vi "Configure Bus.vi"(4 "Digital Channel List":bool[](array[boolean]), 5 "Enable Bus (T: Enable)":bool=TRUE, 6 "Slope (0: Rising)":i32(ring) items=["Rising", "Falling", "Either"], 7 "Bus (51: Bus 1)":i32(ring)=51 items=["Bus 1"=51, "Bus 2"=52, "Bus 3"=53, "Bus 4"=54], 8 "error in (no error)":errorcluster, 9 "Clock Source (19: None)":i32(ring)=19 items=["Channel 1"=1, "Channel 2"=2, "Channel 3"=3, "Channel 4"=4, "DIG 0"=20, "DIG 1"=21, "DIG 2"=22, "DIG 3"=23, "DIG 4"=24, "DIG 5"=25, "DIG 6"=26, "DIG 7"=27, "DIG 8"=28, "DIG 9"=29, "DIG 10"=30, "DIG 11"=31, "DIG 12"=32, "DIG 13"=33, "DIG 14"=34, "DIG 15"=35, "None"=19], 10 "Bus Type (4: XAUI)":i32(ring)=4 items=["Can", "Fibre Channel", "SATA", "SPI", "XAUI", "Flex Ray", "GEN8B10B", "Generic", "IIC", "Infinite Band", "Most", "PCI Express", "SAS", "Hot Link", "MIPI", "DVI", "USB2", "USB3", "UART", "PCI3", "MPHY", "LIN", "JTAG", "GEN8B10B ", "E10GBASEKR", "DDR", "RFFE", "SVID", "CSI3", "Dig Rf", "JESD204B", "LLI", "SSIC", "UFS", "UNI Pro"], 11 "VISA resource name":refnum<visa-resource-name>) -> (0 "error out":errorcluster, 3 "VISA resource name out":refnum<visa-resource-name>)   [LabVIEW 2020, in "Agilent 90000 Series.lvlib"]
doc: "Configures the BUS settings in serial data analysis."
uses:
  Agilent 90000 Series.lvlib
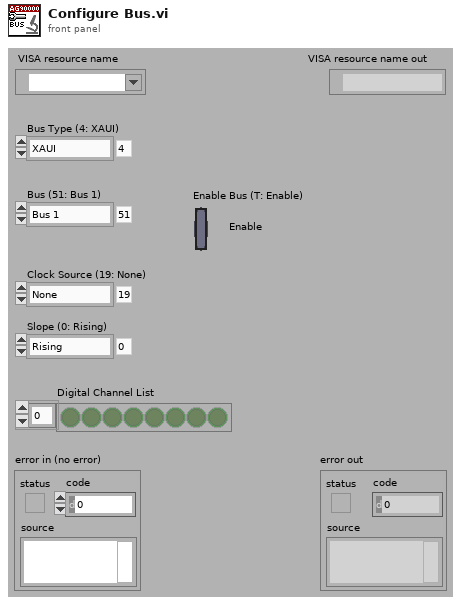
[diagram p1: front panel]
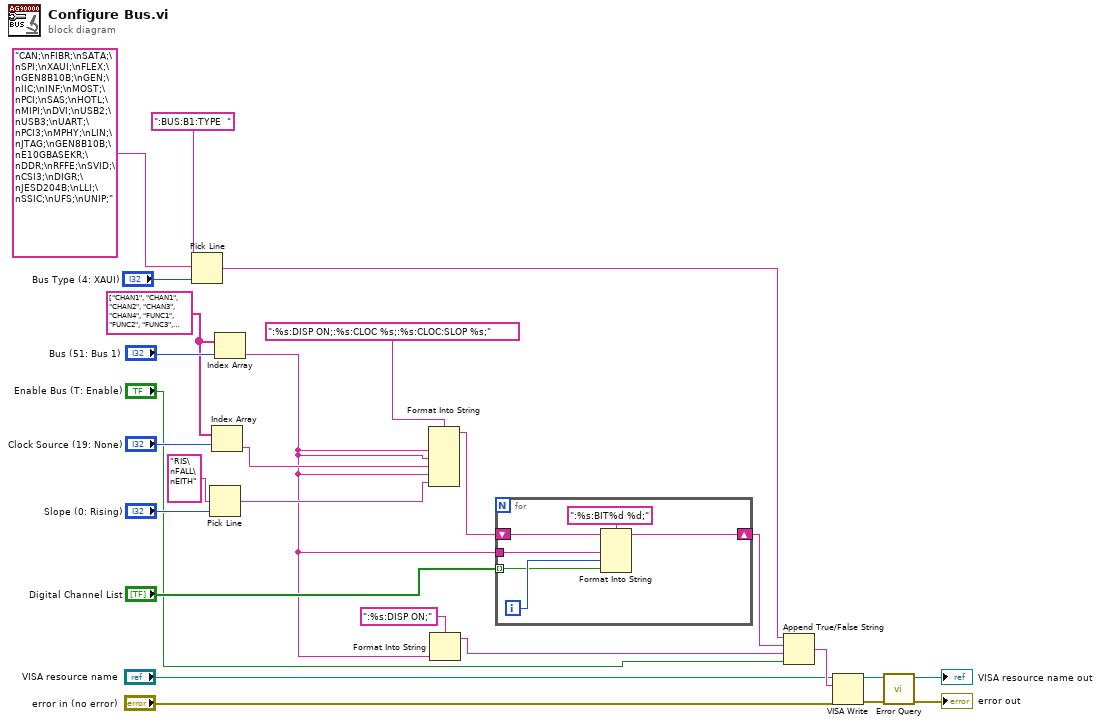
[diagram p0: block diagram]
diagram:
  w17 = string[] ["CHAN1", "CHAN1", "CHAN2", "CHAN3", "CHAN4", "FUNC1", "FUNC2", "FUNC3", "FUNC4", "WMEM1", "WMEM2", "WMEM3", "WMEM4", "AUX", "LINE", "CLOC", "MTR", "MSP", "EQU", "NONE", "DIG0", "DIG1", "DIG2", "DIG3", "DIG4", "DIG5", "DIG6", "DIG7", "DIG8", "DIG9", "DIG10", "DIG11", "DIG12", "DIG13", "DIG14", "DIG15", "", "", "", "", "", "POD1", "POD2", "", "", "", "", "", "", "", "", "BUS1", "BUS2", "BUS3", "BUS4"]
  n1 = Pick Line(string ("")=":BUS:B1:TYPE  ", multi-line string="CAN;\nFIBR;\nSATA;\nSPI;\nXAUI;\nFLEX;\nGEN8B10B;\nGEN;\nIIC;\nINF;\nMOST;\nPCI;\nSAS;\nHOTL;\nMIPI;\nDVI;\nUSB2;\nUSB3;\nUART;\nPCI3;\nMPHY;\nLIN;\nJTAG;\nGEN8B10B;\nE10GBASEKR;\nDDR;\nRFFE;\nSVID;\nCSI3;\nDIGR;\nJESD204B;\nLLI;\nSSIC;\nUFS;\nUNIP;", line index="Bus Type (4: XAUI)") -> (output string=w4:string)
  n2 = Pick Line(multi-line string="RIS\nFALL\nEITH", line index="Slope (0: Rising)") -> (output string=w12:string)  [unwired: 1 out]
  n3 = Index Array(array=w17, index="Clock Source (19: None)") -> (element=w13:string)
  n4 = Index Array(array=w17, index="Bus (51: Bus 1)") -> (element=w6:string)
  n5 = Format Into String(format string=":%s:DISP ON;:%s:CLOC %s;:%s:CLOC:SLOP %s;", w6, w6, w13, w6, w12) -> (resulting string=w10:string)  [unwired: 2 in, 1 out]
  n6 = Format Into String(format string=":%s:DISP ON;", w6) -> (resulting string=w5:string)  [unwired: 2 in, 1 out]
  n7 = for {
    tunnel: "Digital Channel List" -> [w30] mode=indexing
    tunnel: w6 -> [w29]
    shift-right: [w27] -> w8
    shift-left: w10 -> [w28]
    i -> [w31]
    n8 = Format Into String(format string=":%s:BIT%d %d;", initial string=w28, w29, w31, w30) -> (resulting string=w27:string)  [unwired: 1 in, 1 out]
  }
  n9 = Append True/False String(1:"Enable Bus (T: Enable)", 2:w5, 3:w8, 4:w4) -> (0:w9:string)
  n10 = VISA Write(VISA resource name="VISA resource name", write buffer=w9, error in (no error)="error in (no error)") -> (VISA resource name out=w24:refnum<visa-resource-name>, error out=w23:errorcluster)  [unwired: 1 out]
  n11 = call "Error Query.vi"("error in (no error)"=w23, "VISA resource name"=w24) -> ("error out"=→"error out":errorcluster, "VISA resource name out"=→"VISA resource name out":refnum<visa-resource-name>)  [unwired: 8 out]
